vi "全局小变量.vi"() -> ()   [LabVIEW 2016]
panel:
  out "F(Flow)ml/min":string
  out "R(Gas)mv":string
  out "P（eq)mv":string
  out "T(cool)℃":string
  out "多位阀的位置":string
  out "数据采集时间间隔":i32
  out "数组大小":i32
  out "跳转次数变量":i32=2
  out "当前步骤":i32
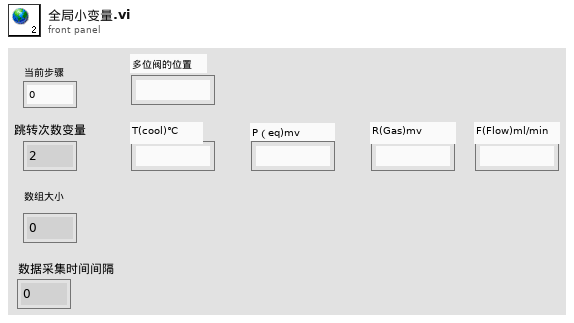
[diagram p1: front panel]
diagram:
